vi "NormalNoRefs.vi"(5 "error in (no error)":errorcluster) -> (19 "error out":errorcluster)   [LabVIEW 2020, in "G#MethodTemplates.lvclass"]
uses:
  G#MethodTemplates.lvclass
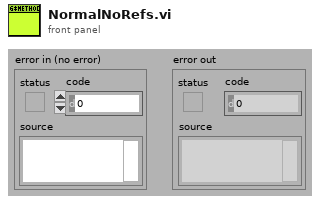
[diagram p1: front panel]
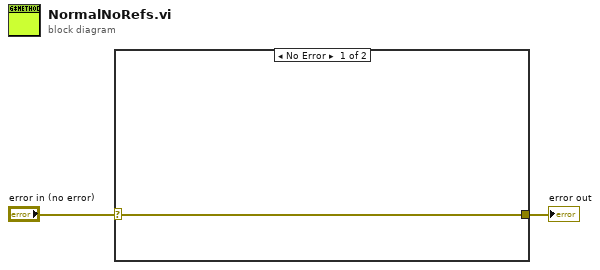
[diagram p0: block diagram]
diagram:
  n1 = case shown="No Error" "error in (no error)" {
    selector: "error in (no error)" -> [w3 w4]
    tunnel: [w3 w4] -> w1
    frame No Error {
    }
    frame Error {
    }
  }
  "error out" <- w1
